vi "generate table.vi"(7 "table":T1, 8 "error in":errorcluster, 10 "engine configuration":refnum<class "engine configuration.lvclass">, 11 "tag bus configurable plugin module configuration":refnum<class "Modbus Slave configuration.lvclass">) -> (0 "error out":errorcluster)   [LabVIEW 2013, in "Modbus Slave editor node.lvclass"]
doc: "Platypus Framework 1.0.1.65\nNI Systems Engineering - National Instruments"
uses:
  Modbus Slave editor node.lvclass
  table reference.ctl
  module/configuration/Modbus Slave configuration.lvclass
  <vilib>/NI/Module Execution Interface/Engine Configuration/engine configuration.lvclass
  <vilib>/NI/Configuration Framework/serializable configuration/NISE_CEF_serializable configuration.lvclass/NISE_CEF_serializable configuration.ctl
  <vilib>/NI/Configuration Framework/serializable configuration/NISE_CEF_serializable configuration.lvclass
  module/configuration/Modbus Slave configuration.lvclass/Modbus Slave configuration.ctl
  table line.ctl
  module/module channel/Modbus Module Channel.lvclass
  <vilib>/NI/Tag Bus/tag/tag descriptor.lvclass/tag descriptor.ctl
  <vilib>/NI/Tag Bus/tag/read tag name.vi
  <vilib>/NI/Configuration Framework/serializable configuration/Read UID.vi
  module/configuration/Read modbus channels.vi
  <vilib>/NI/Tag Bus/tag/tag descriptor.lvclass
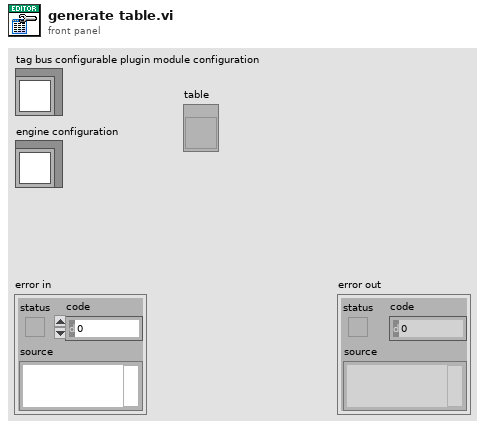
[diagram p1: front panel]
types:
  T1 = typedef "Modbus Slave editor node.lvclass/table reference.ctl" = refnum<vi>
  T2 = typedef "Modbus Slave editor node.lvclass/table line.ctl" = cluster{"mbchan":refnum<class "Modbus Module Channel.lvclass">, "tag name":string}
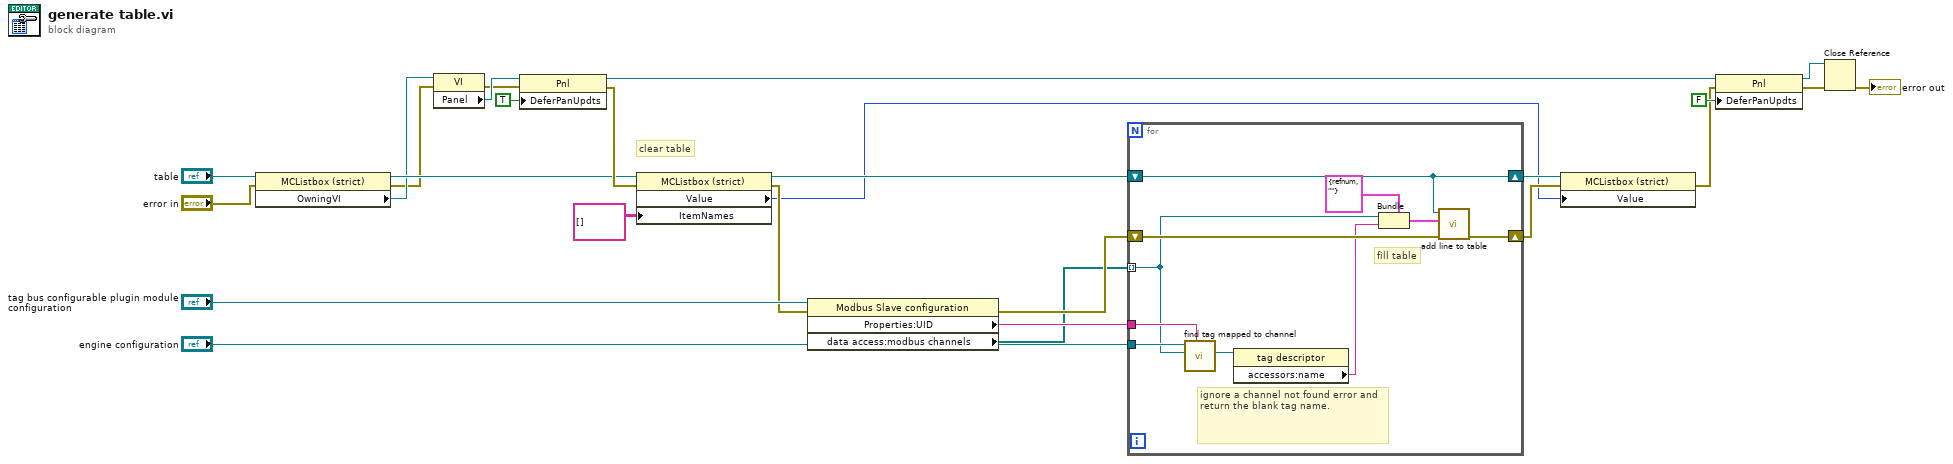
[diagram p0: block diagram]
diagram:
  # "clear table"
  n1 = property class="MCListbox (strict)"(reference="table", error in="error in") -> (reference out=w7:T1, error out=w4:errorcluster, "OwningVI"=w5:refnum<vi>)
  n2 = property class="VI"(reference=w5, error in=w4) -> (error out=w13:errorcluster, "Panel"=w14:refnum<vi>)  [unwired: 1 out]
  n3 = property class="Pnl"(reference=w14, error in=w13, "DeferPanUpdts"=TRUE ("Defer Panel Updates")) -> (reference out=w10:refnum<vi>, error out=w12:errorcluster)
  n4 = property class="MCListbox (strict)"(reference=w7, error in=w12, "ItemNames"=string[][] [] ("Item Names")) -> (reference out=w25:T1, error out=w21:errorcluster, "Value"=w16:i32)
  n5 = property class="Modbus Slave configuration"(reference="tag bus configurable plugin module configuration", error in=w21) -> (error out=w20:errorcluster, "Properties:UID"=w22:string, "data access:modbus channels"=w1:refnum<class "Modbus Module Channel.lvclass">[])  [unwired: 1 out]
  n6 = for {
    shift-right: [w36] -> w17
    shift-left: w20 -> [w33]
    tunnel: w1 -> [w30] mode=indexing
    tunnel: "engine configuration" -> [w32]
    tunnel: w22 -> [w31]
    shift-right: [w27] -> w18
    shift-left: w25 -> [w27]
    # "ignore a channel not found error and return the blank tag name."
    # "fill table"
    n7 = call <vilib>:"find tag mapped to channel.vi"("owner"=w31, "channel"=w30, "engine configuration in"=w32) -> ("tag"=w29:refnum<class "tag descriptor.lvclass">)  [unwired: 6 in, 2 out]
    n8 = property class="tag descriptor"(reference=w29) -> ("accessors:name"=w28:string)  [unwired: 1 in, 2 out]
    n9 = Bundle(cluster=T2 {"mbchan"=refnum, "tag name"=""} ("line"), "mbchan"=w30, "tag name"=w28) -> (w34:T2)
    n10 = call "add line to table.vi"("error in"=w33, "line"=w34, "operations table"=w27) -> ("error out"=w36:errorcluster)  [unwired: 8 in]
  }
  n11 = property class="MCListbox (strict)"(reference=w18, error in=w17, "Value"=w16) -> (error out=w9:errorcluster)  [unwired: 1 out]
  n12 = property class="Pnl"(reference=w10, error in=w9, "DeferPanUpdts"=FALSE ("Defer Panel Updates")) -> (reference out=w2:refnum<vi>, error out=w8:errorcluster)
  n13 = Close Reference(reference=w2, error in (no error)=w8) -> (error out=→"error out":errorcluster)
